vi "deinitialize.vi"(0 "HGF_DSCEvent":refnum<class "HGF_DSCEvent.lvclass">, 5 "error in (no error)":errorcluster) -> (19 "error out":errorcluster)   [LabVIEW 2012, in "HGF_DSC.lvlib" / "HGF_DSCEvent.lvclass"]
doc: "This is a dynamic dispatch VI. It can be overwritten by childclasses to release allocated recources."
uses:
  HGF_DSCEvent.lvclass
  HGF_DSCEvent.lvclass/HGF_DSCEvent.ctl
  HGF_SV/HGF_SVEvent/HGF_SVEvent.lvclass
  HGF_DSCCommand/HGF_DSCCommand.lvclass
  HGF_DSCFactory/HGF_DSCFactory.lvclass
  HGF_BaseClasses/HGF_Event/HGF_Event.lvclass
  HGF_DSCSubscriber/HGF_DSCSubscriber.lvclass
  HGF_BaseClasses/HGF_NetworkEvent/HGF_NetworkEvent.lvclass/HGF_NetworkEvent.lvclass
  HGF_BaseClasses/HGF_NetworkVisitor/HGF_NetworkVisitor.lvclass
  HGF_BaseClasses/HGF_Factory/HGF_Factory.lvclass
  HGF_SV/Visitors/HGF_SVMonitorVisitor_deregister/HGF_SVMonitorVisitor_deregister.lvclass
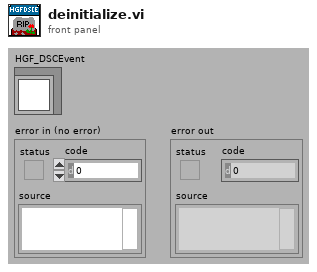
[diagram p1: front panel]
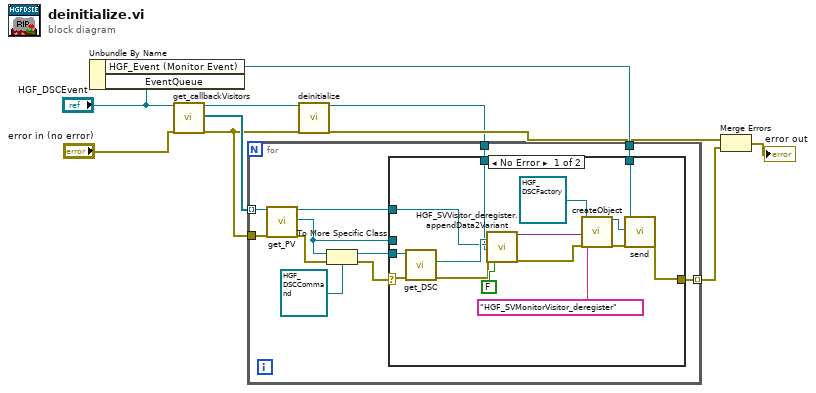
[diagram p0: block diagram]
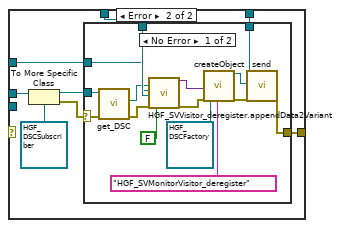
[diagram p2: hidden frame]
diagram:
  n1 = Unbundle By Name("HGF_DSCEvent") -> ("HGF_Event (Monitor Event)"=w8:refnum<class "HGF_Event.lvclass">)  [unwired: 1 out]
  n2 = call "get_callbackVisitors.vi"("HGF_NetworkEvent"="HGF_DSCEvent", "error in (no error)"="error in (no error)") -> ("dup HGF_NetworkEvent"=w1:refnum<class "HGF_DSCEvent.lvclass">, "callbackVisitors"=w7:refnum<class "HGF_NetworkVisitor.lvclass">[], "error out"=w2:errorcluster)  [unwired: 15 out]
  n3 = for {
    tunnel: w7 -> [w20] mode=indexing
    tunnel: [w16] -> w6 mode=indexing
    tunnel: w2 -> [w12]
    tunnel: w8 -> [w11]
    tunnel: w1 -> [w10]
    n4 = call "get_PV.vi"("HGF_NetworkData"=w20, "error in (no error)"=w12) -> ("dup HGF_NetworkData"=w17:refnum<class "HGF_NetworkVisitor.lvclass">, "HGV_PVBase"=w13:refnum<class "HGF_PVBase.lvclass">, "error out"=w14:errorcluster)  [unwired: 15 out]
    n5 = To More Specific Class(target class=refnum<class "HGF_DSCCommand.lvclass"> refnum ("DSC.lvlib:HGF_DSCCommand.lvclass"), reference=w13, error in=w14) -> (specific class reference=w18:refnum<class "HGF_DSCCommand.lvclass">, error out=w19:errorcluster)
    n6 = case shown="No Error" w19 {
      selector: w19 -> [w34 _]
      tunnel: w18 -> [w35 _]
      tunnel: w17 -> [w25 w41]
      tunnel: [w32 w40] -> w16
      tunnel: w13 -> [_ w38]
      tunnel: w11 -> [w31 w37]
      tunnel: w10 -> [w21 w36]
      frame No Error {
        n7 = call-dynamic "get_DSC.vi"("error in (no error)"=w34, "HGF_DSCCommand.lvclass in"=w35) -> ("error out"=w22:errorcluster, "SV"=w26:refnum<k21>)  [unwired: 8 out]
        n8 = call "HGF_SVVisitor_deregister.appendData2Variant.vi"("Shared Variable Control (DSC)"=w26, "HGF_NetworkVisitor"=w25, "HGF_TriggeredEvent"=w21, "error in"=w22, "Rem SV/Visitor from List"=FALSE) -> ("dup variant"=w27:variant, "error out"=w23:errorcluster)  [unwired: 13 in]
        n9 = call "createObject.vi"("HGF_Factory"=refnum<class "HGF_DSCFactory.lvclass"> refnum ("DSC.lvlib:HGF_DSCFactory.lvclass"), "initializationData"=w27, "error in (no error)"=w23, "className"="HGF_SVMonitorVisitor_deregister") -> ("HGF_Object"=w30:refnum<class "HGF_Factory.lvclass">, "error out"=w33:errorcluster)  [unwired: 13 in, 1 out]
        n10 = call-dynamic "send.vi"("HGF_Event"=w31, "Object"=w30, "error in (no error)"=w33) -> ("error out"=w32:errorcluster)  [unwired: 14 in, 2 out]
      }
      frame Error {
        n11 = To More Specific Class(target class=refnum<class "HGF_DSCSubscriber.lvclass"> refnum ("DSC.lvlib:HGF_DSCSubscriber.lvclass"), reference=w38) -> (specific class reference=w42:refnum<class "HGF_DSCSubscriber.lvclass">, error out=w43:errorcluster)  [unwired: 1 in]
        n12 = case shown="No Error" w43 {
          selector: w43 -> [w57 w59]
          tunnel: w42 -> [w58 _]
          tunnel: w41 -> [w45 _]
          tunnel: [w53 w59] -> w40
          tunnel: w37 -> [w51 _]
          tunnel: w36 -> [w46 _]
          frame No Error {
            n13 = call "get_DSC.vi"("error in (no error)"=w57, "HGF_DSCSubscriber.lvclass in"=w58) -> ("error out"=w47:errorcluster, "Shared Variable"=w44:refnum<k21>)  [unwired: 8 out]
            n14 = call "HGF_SVVisitor_deregister.appendData2Variant.vi"("Shared Variable Control (DSC)"=w44, "HGF_NetworkVisitor"=w45, "HGF_TriggeredEvent"=w46, "error in"=w47, "Rem SV/Visitor from List"=FALSE ("Switch")) -> ("dup variant"=w50:variant, "error out"=w49:errorcluster)  [unwired: 13 in]
            n15 = call "createObject.vi"("HGF_Factory"=refnum<class "HGF_DSCFactory.lvclass"> refnum ("DSC.lvlib:HGF_DSCFactory.lvclass"), "initializationData"=w50, "error in (no error)"=w49, "className"="HGF_SVMonitorVisitor_deregister") -> ("HGF_Object"=w52:refnum<class "HGF_Factory.lvclass">, "error out"=w54:errorcluster)  [unwired: 13 in, 1 out]
            n16 = call-dynamic "send.vi"("HGF_Event"=w51, "Object"=w52, "error in (no error)"=w54) -> ("error out"=w53:errorcluster)  [unwired: 14 in, 2 out]
          }
          frame Error {
          }
        }
      }
    }
  }
  n17 = call-parent "deinitialize.vi"("HGF_SVEvent"=w1, "error in (no error)"=w2) -> ("error out"=w5:errorcluster)  [unwired: 17 out]
  n18 = Merge Errors(w5, w6) -> (→"error out":errorcluster)
